vi "MoveSelection.vi"(8 "error in (no error)":errorcluster, 10 "Engine in":refnum<class "Engine.lvclass">, 11 "Menu in":refnum<class "Menu.lvclass">) -> (0 "error out":errorcluster, 1 "Changed?":bool, 2 "Engine out":refnum<class "Engine.lvclass">, 3 "Menu out":refnum<class "Menu.lvclass">)   [LabVIEW 2019, in "RT_Game.lvlib" / "Menu.lvclass"]
uses:
  Menu.lvclass
  C:/Users/FreshBob/Dropbox/VIs/myRIO_GameConsole/RT/RT_Game/Game/Game.lvclass
  Engine/Engine.lvclass
  Engine/Engine.lvclass/Engine.ctl
  Cursor/Cursor.lvclass
  C:/Users/FreshBob/Dropbox/VIs/myRIO_GameConsole/RT/RT_Game/RT_Sprite/RT_Sprite.lvclass
  Game/Game.lvclass/Game.ctl
  Cursor/Cursor.lvclass/Cursor.ctl
  Menu.lvclass/Menu.ctl
  Game/Read Sprite1.vi
  Cursor/Read selection.vi
  Game/Write Sprite1.vi
  RT_Sprite/RT_Sprite.lvclass
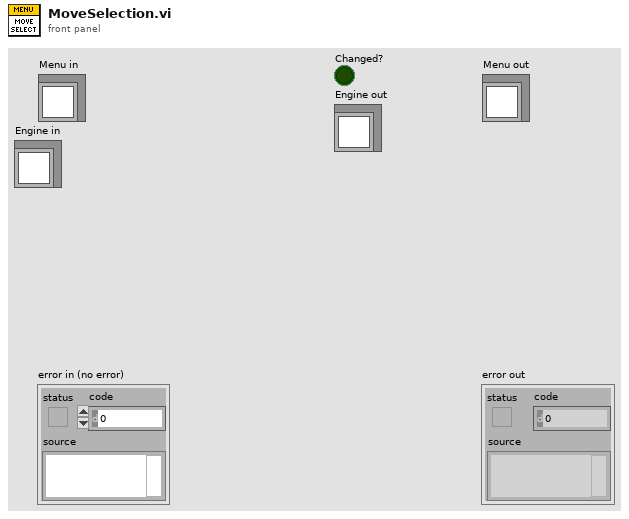
[diagram p1: front panel]
types:
  T1 = typedef "RT_Game.lvlib/Game.lvclass/Controls.ctl" = cluster{"Controls_1":T2, "Controls_2":cluster{"DirectionX":i8, "DirectionY":i8, "Button1":bool, "Button2":bool}, "SystemButton":bool}
  T2 = typedef "RT_Game.lvlib/Game.lvclass/ControlPlayer.ctl" = cluster{"DirectionX":i8, "DirectionY":i8, "Button1":bool, "Button2":bool}
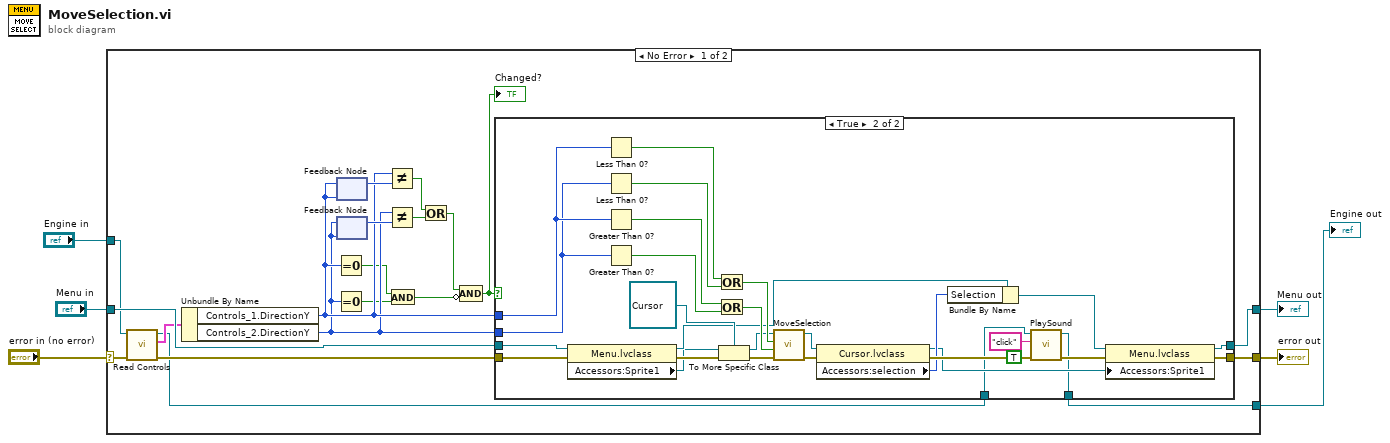
[diagram p0: block diagram]
diagram:
  n1 = case shown="No Error" "error in (no error)" {
    selector: "error in (no error)" -> [w14 w61]
    tunnel: [w13 w61] -> w5
    tunnel: [w12 w60] -> w3
    tunnel: "Menu in" -> [w15 w60]
    tunnel: "Engine in" -> [w9 w59]
    tunnel: [w7 w59] -> w1
    frame No Error {
      n2 = call "Read Controls.vi"("error in (no error)"=w14, "Engine in"=w9) -> ("error out"=w11:errorcluster, "Controls"=w10:T1, "Engine out"=w8:refnum<class "Engine.lvclass">)  [unwired: 7 in]
      n3 = Unbundle By Name(w10) -> ("Controls_1.DirectionY"=w21:i8, "Controls_2.DirectionY"=w20:i8)
      n4 = Equal To 0?(x=w21) -> (x = 0?=w19:bool)
      n5 = Equal To 0?(x=w20) -> (x = 0?=w18:bool)
      n6 = feedback-in #1(w21) -> ()
      n7 = feedback #1(w21) -> (w26:i8)
      n8 = feedback #2(w20) -> (w25:i8)
      n9 = feedback-in #2(w20) -> ()
      n10 = Not Equal?(x=w21, y=w26) -> (x != y?=w24:bool)
      n11 = Not Equal?(x=w20, y=w25) -> (x != y?=w23:bool)
      n12 = And(x=w19, y=w18) -> (x .and. y?=w16:bool)
      n13 = Or(x=w24, y=w23) -> (x .or. y?=w22:bool)
      n14 = Compound Arithmetic op=AND(w22, invert w16) -> (w17:bool)
      "Changed?" <- w17
      n15 = case shown="True" w17 {
        tunnel: [w29 w36] -> w12
        tunnel: w21 -> [_ w58]
        tunnel: w20 -> [_ w57]
        tunnel: [w28 w35] -> w13
        tunnel: w15 -> [w29 w43]
        tunnel: w11 -> [w28 w42]
        tunnel: w8 -> [w27 w31]
        tunnel: [w27 w30] -> w7
        frame False {
        }
        frame True {
          n16 = property class="Menu.lvclass"(reference=w43, error in=w42) -> (reference out=w41:refnum<class "Menu.lvclass">, error out=w40:errorcluster, "Accessors:Sprite1"=w39:refnum<class "RT_Sprite.lvclass">)
          n17 = Less Than 0?(x=w58) -> (x < 0?=w52:bool)
          n18 = Less Than 0?(x=w57) -> (x < 0?=w53:bool)
          n19 = Greater Than 0?(x=w58) -> (x > 0?=w55:bool)
          n20 = Greater Than 0?(x=w57) -> (x > 0?=w54:bool)
          n21 = Or(x=w52, y=w53) -> (x .or. y?=w50:bool)
          n22 = Or(x=w55, y=w54) -> (x .or. y?=w51:bool)
          n23 = To More Specific Class(target class=refnum<class "Cursor.lvclass"> refnum ("Cursor in"), reference=w39, error in=w40) -> (specific class reference=w47:refnum<class "Cursor.lvclass">, error out=w49:errorcluster)
          n24 = call "MoveSelection.vi"("error in (no error)"=w49, "down?"=w51, "up?"=w50, "Cursor in"=w47) -> ("error out"=w56:errorcluster, "Cursor out"=w45:refnum<class "Cursor.lvclass">)  [unwired: 6 in]
          n25 = property class="Cursor.lvclass"(reference=w45, error in=w56) -> (reference out=w37:refnum<class "Cursor.lvclass">, error out=w46:errorcluster, "Accessors:selection"=w44:i16)
          n26 = Bundle By Name(cluster=w41, "Selection"=w44) -> (w32:refnum<class "Menu.lvclass">)
          n27 = call "PlaySound.vi"("error in (no error)"=w46, "Overwrite"=TRUE, "Name"="click", "Engine in"=w31) -> ("error out"=w38:errorcluster, "Engine out"=w30:refnum<class "Engine.lvclass">)  [unwired: 6 in]
          n28 = property class="Menu.lvclass"(reference=w32, error in=w38, "Accessors:Sprite1"=w37) -> (reference out=w36:refnum<class "Menu.lvclass">, error out=w35:errorcluster)
        }
      }
    }
    frame Error {
    }
  }
  "error out" <- w5
  "Menu out" <- w3
  "Engine out" <- w1
